vi "Vision Research Phantom Series PhFile PhWriteCineFile.vi"(1 "CH in":u32, 5 "Error In (no error)":errorcluster, 7 "CallID":u32) -> (15 "CH out":u32, 19 "Error Out":errorcluster)   [LabVIEW 2013, in "VRI.lvlib"]
doc: "PhFile.dll\n\nPhWriteCineFile\nHRESULT PhWriteCineFile(CINEHANDLE CH, PROGRESSCB pfnCallback);\n\nParameters Description\nCH(in) Handle of the cine to be saved.\nCallID (in) Choose a CallID(unsigned int <= 15) and pass it in the \n place of the Function pointer parameter.\n To retrieve progress information for that call, you must \n call LVProgress with chosen CallID within a loop. The time \n consuming call and the LVProgress call must be in separate \n threads.\nReturn HRESULT (0 = Ok)\nComments This function saves the cine, represented by the cine \n handle CH. You must call PhGetSaveCineName before this.\n\nWritten by:\nBLOOMY CONTROLS, INC\nWINDSOR, CT 06095, USA\n860-298-9925\nwww.bloomy.com\nV1.0.0\nMay, 2004"
uses:
  VRI.lvlib
  Phantom DLLs/PhFile.Dll
panel:
  # "For instructions on the use of this VI, press Ctrl+H to display the help window and move the mouse over the icon, controls, and indicators"
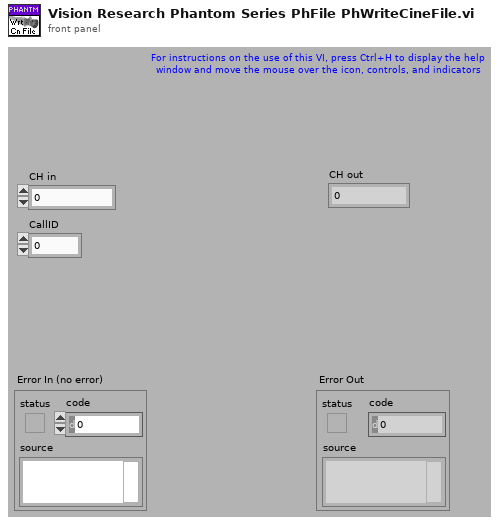
[diagram p1: front panel]
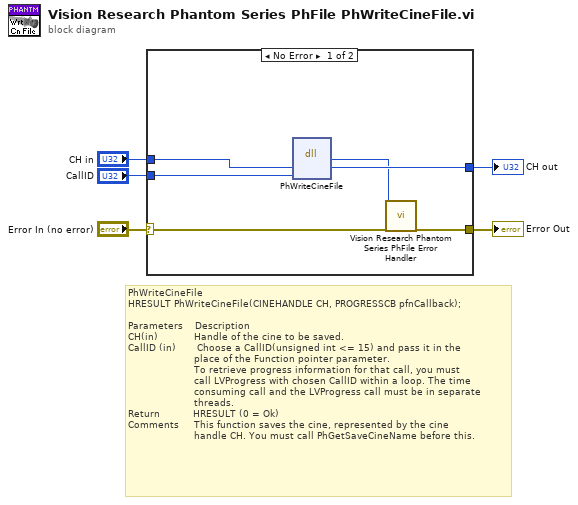
[diagram p0: block diagram]
diagram:
  # "PhWriteCineFile\nHRESULT PhWriteCineFile(CINEHANDLE CH, PROGRESSCB pfnCallback);\n\nParameters    Description\nCH(in)            Handle of the cine to be saved.\nCallID (in)       Choose a CallID(unsigned int <= 15) and pass it in the \n                      place of the Function pointer parameter.\n                      To retrieve progress information for that call, you must \n                      call LVProgress with chosen CallID within a loop. The time \n                      consuming call and the LVProgress call must be in separate \n                      threads.\nReturn           HRESULT (0 = Ok)\nComments     This function saves the cine, represented by the cine \n                      handle CH. You must call PhGetSaveCineName before this."
  n1 = case shown="No Error" "Error In (no error)" {
    selector: "Error In (no error)" -> [w11 w13]
    tunnel: [w10 w13] -> w4
    tunnel: "CallID" -> [w9 _]
    tunnel: "CH in" -> [w8 w12]
    tunnel: [w7 w12] -> w1
    frame No Error {
      n2 = dll-call lib="C:/Projects/SDK/64-bit/Vision Research Phantom Series Labview Driver/Phantom DLLs/PhFile.dll" fn="PhWriteCineFile"("CH"=w8, "CallID"=w9) -> ("HRESULT"=w6:i32, "CH"=w7:u32)  [unwired: 4 in, 2 out]
      n3 = call "Vision Research Phantom Series PhFile Error Handler.vi"("Error Code (0)"=w6, "Error In (no error)"=w11) -> ("Error Out"=w10:errorcluster)  [unwired: 17 out]
    }
    frame Error {
    }
  }
  "Error Out" <- w4
  "CH out" <- w1
